vi "HumanActionCache.vi"(6 "State":i32, 7 "Rotation":dbl, 8 "Right X":dbl, 9 "Right Y":dbl, 10 "Left X":dbl, 11 "Left Y":dbl) -> (1 "AMotorDemand":dbl, 2 "YMotorDemand":dbl, 3 "XMotorDemand":dbl)   [LabVIEW 2023]
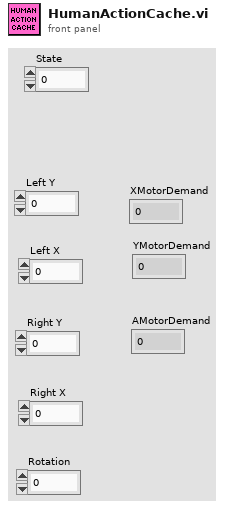
[diagram p1: front panel]
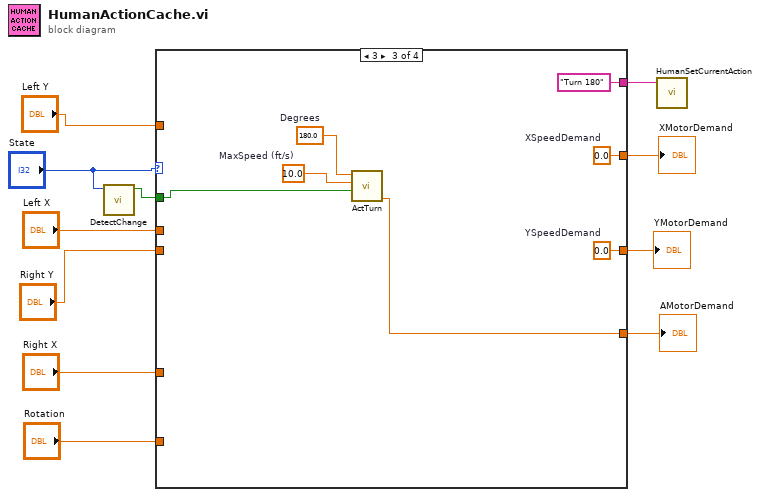
[diagram p0: block diagram]
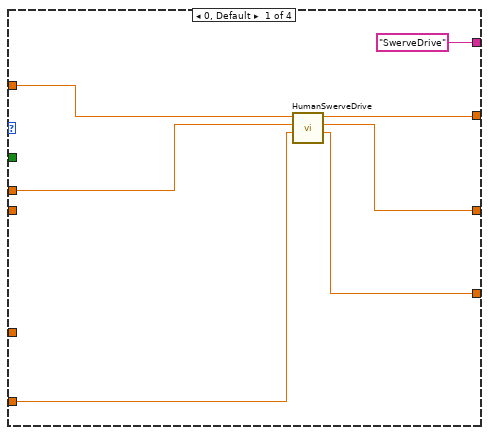
[diagram p2: hidden frame]
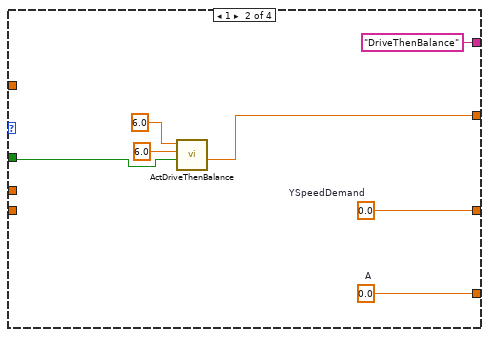
[diagram p3: hidden frame]
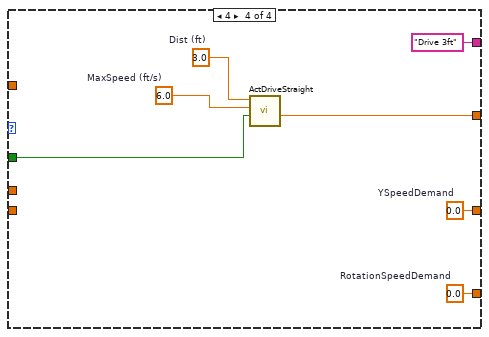
[diagram p4: hidden frame]
diagram:
  n1 = call "DetectChange.vi"("Value"="State") -> ("Changed"=w5:bool)  [unwired: 10 in]
  n2 = case shown="3" "State" {
    tunnel: "Left Y" -> [w17 _ _ _]
    tunnel: "Right X" -> [_ _ _ _]
    tunnel: [w14 w25 w26 w38] -> w9
    tunnel: [w13 w20 w27 w37] -> w8
    tunnel: "Right Y" -> [_ _ _ _]
    tunnel: w5 -> [_ w22 w31 w33]
    tunnel: ["SwerveDrive" "DriveThenBalance" "Turn 180" "Drive 3ft"] -> w4
    tunnel: "Left X" -> [w16 _ _ _]
    tunnel: "Rotation" -> [w15 _ _ _]
    tunnel: [w12 w19 w28 w36] -> w1
    frame 0, Default {
      n3 = call "HumanSwerveDrive.vi"("Rotation"=w15, "Y"=w16, "X"=w17) -> ("A"=w12:dbl, "Y"=w13:dbl, "X"=w14:dbl)  [unwired: 6 in]
    }
    frame 1 {
      w19 = 0.0  # A
      w20 = 0.0  # YSpeedDemand
      n4 = call "ActDriveThenBalance.vi"("FirstTime"=w22, "MaxSpeed (ft/s)"=6.0, "Dist (ft)"=6.0) -> ("XSpeedDemand"=w25:dbl)  [unwired: 7 in, 1 out]
    }
    frame 3 {
      w26 = 0.0  # XSpeedDemand
      w27 = 0.0  # YSpeedDemand
      w29 = 180.0  # Degrees
      w30 = 10.0  # MaxSpeed (ft/s)
      n5 = call "ActTurn.vi"("FirstTime"=w31, "MaxSpeed (ft/s)"=w30, "Degrees"=w29) -> ("RotationSpeedDemand Deg/Sec"=w28:dbl)  [unwired: 7 in, 1 out]
    }
    frame 4 {
      w34 = 6.0  # MaxSpeed (ft/s)
      w35 = 3.0  # Dist (ft)
      w36 = 0.0  # RotationSpeedDemand
      w37 = 0.0  # YSpeedDemand
      n6 = call "ActDriveStraight.vi"("FirstTime"=w33, "MaxSpeed (ft/s)"=w34, "Dist (ft)"=w35) -> ("XSpeedDemand"=w38:dbl)  [unwired: 7 in, 1 out]
    }
  }
  "XMotorDemand" <- w9
  "YMotorDemand" <- w8
  "AMotorDemand" <- w1
  n7 = call "HumanSetCurrentAction.vi"("CurrentState"=w4) -> ()  [unwired: 11 in]
